vi "圆柱体体积.vi"(8 "Height":dbl, 11 "Radious":dbl) -> (3 "Area":dbl=nan)   [LabVIEW 2012]
doc: "功能：\n计算圆柱体体积。\n\n公式：\n\nV=底面积*高\n\ncsxcs_366创建"
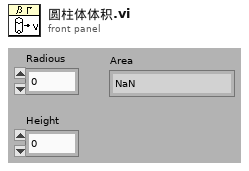
[diagram p1: front panel]
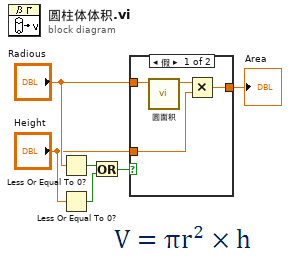
[diagram p0: block diagram]
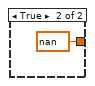
[diagram p2: hidden frame]
diagram:
  n1 = Less Or Equal To 0?(x="Radious") -> (x <= 0?=w6:bool)
  n2 = Less Or Equal To 0?(x="Height") -> (x <= 0?=w5:bool)
  n3 = Or(x=w6, y=w5) -> (x .or. y?=w4:bool)
  n4 = case shown="假" w4 {
    tunnel: [w7 nan ("t")] -> w3
    tunnel: "Radious" -> [w9 _]
    tunnel: "Height" -> [w8 _]
    frame False {
      n5 = call "圆面积.vi"("Radious"=w9) -> ("Area"=w10:dbl)  [unwired: 10 in]
      n6 = Multiply(x=w10, y=w8) -> (x*y=w7:dbl)
    }
    frame True {
    }
  }
  "Area" <- w3
